vi "RefreshTableName.vi"(8 "error in (no error)":errorcluster, 10 "TableName":string[](array[string]), 11 "DataBase in":refnum<class "DataBase.lvclass">) -> (0 "error out":errorcluster, 3 "DataBase out":refnum<class "DataBase.lvclass">)   [LabVIEW 2019, in "DataBase.lvlib" / "DataBase.lvclass"]
uses:
  DataBase.lvclass
  DataBase.lvclass/DataBase.ctl
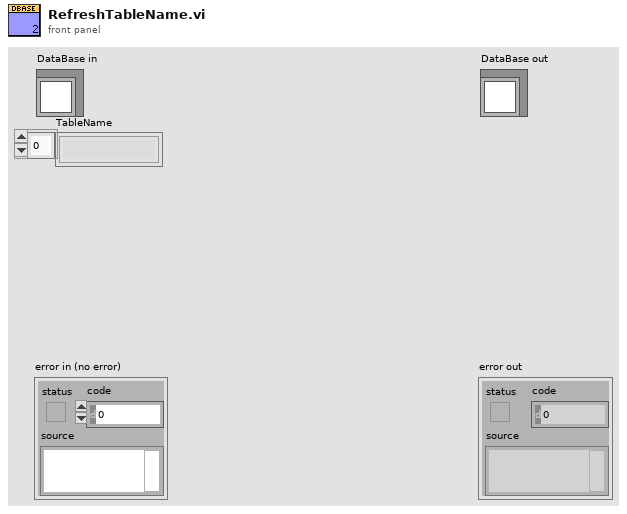
[diagram p1: front panel]
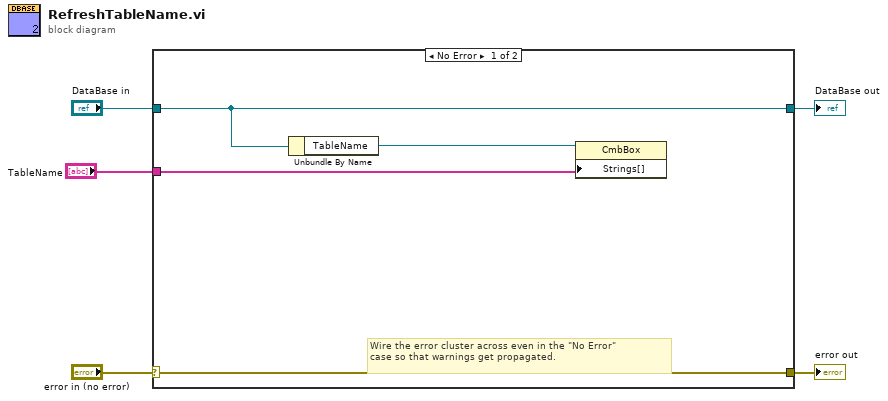
[diagram p0: block diagram]
diagram:
  n1 = case shown="No Error" "error in (no error)" {
    selector: "error in (no error)" -> [w9 w11]
    tunnel: [w9 w11] -> w4
    tunnel: [w8 w10] -> w2
    tunnel: "DataBase in" -> [w8 w10]
    tunnel: "TableName" -> [w6 _]
    frame No Error {
      # "Wire the error cluster across even in the \"No Error\"\ncase so that warnings get propagated."
      n2 = Unbundle By Name(w8) -> ("TableName"=w7:refnum<vi>)
      n3 = property class="CmbBox"(reference=w7, "Strings[]"=w6) -> ()  [unwired: 1 in, 2 out]
    }
    frame Error {
    }
  }
  "error out" <- w4
  "DataBase out" <- w2
